vi "VFH-read_file-R140_waterfile.vi"(8 "error in (no error)":errorcluster) -> (0 "error out":errorcluster, 2 "Array":T1[](array[typedef]))   [LabVIEW 2020, in "VFH-VNA_File_Handler.lvlib"]
uses:
  VFH-VNA_File_Handler.lvlib
  VFH-file_cluster-r140_water.ctl
  <vilib>/addons/_office/excel.llb/Excel Get Data ([dbl]).vi
  <vilib>/Utility/NIReport.llb/NI_report.lvclass
  <vilib>/Utility/NIReport.llb/Excel/NI_Excel.lvclass
  <vilib>/addons/_office/NI_ReportGenerationToolkit.lvlib
panel:
  out "XY Graph":cluster{"Frequency":dbl[], "Permativity'":dbl[]}(graph)
  out "handled Data":dbl[](array[numeric])
  out "Waveform Graph 2":dbl[](graph)
  out "Waveform Graph":dbl[](graph)
  out "Sheet 1 Data":dbl[][](array[numeric]) format="%.2f"
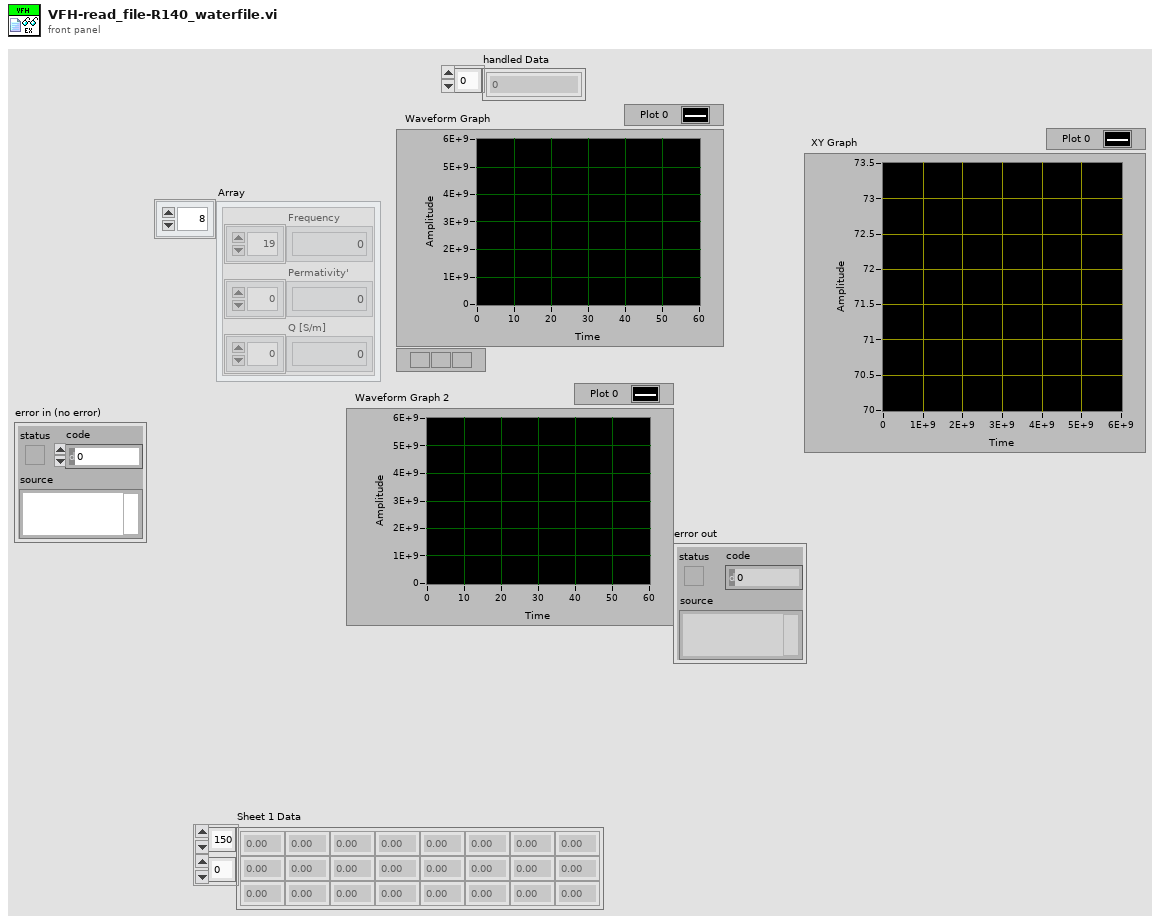
[diagram p1: front panel]
types:
  T1 = typedef "VFH-VNA_File_Handler.lvlib/VFH-file_cluster-r140_water.ctl" = cluster{"Frequency":dbl[], "Permativity'":dbl[], "Q [S/m]":dbl[]}
  T2 = enum16{"Standard Report", "HTML", "Word", "Excel"}
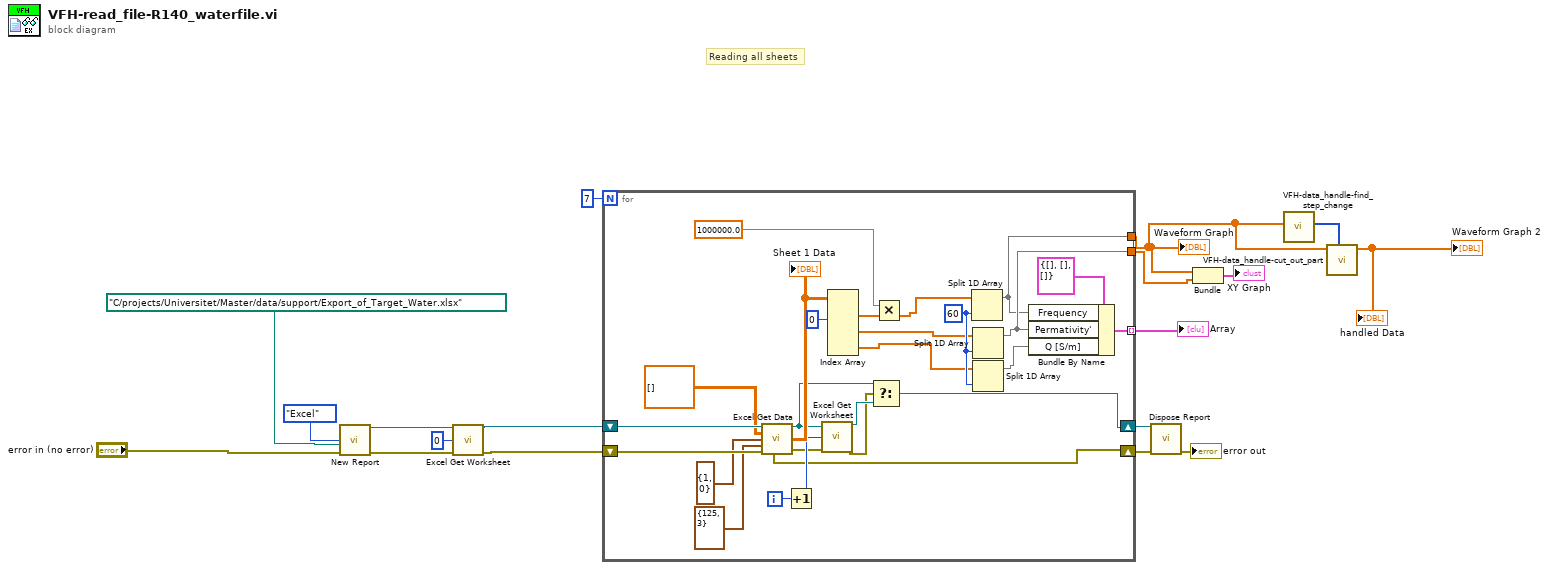
[diagram p0: block diagram]
diagram:
  # "Reading all sheets"
  n1 = call <vilib>:"New Report.vi"("report type"=T2."Excel", "template (empty)"=path "C:/projects/Universitet/Master/data/support/Export_of_Target_Water.xlsx" ("file path (dialog if empty)"), "error in (no error)"="error in (no error)") -> ("report out"=w12:refnum<class "NI_report.lvclass">, "error out"=w11:errorcluster)  [unwired: 3 in, 8 out]
  n2 = call <vilib>:"Excel Get Worksheet.vi"("report in"=w12, "worksheet index (0)"=0, "error in (no error)"=w11) -> ("report out"=w9:refnum<class "NI_report.lvclass">, "error out"=w8:errorcluster)  [unwired: 11 out]
  n3 = for {
    N: 7 -> [_]
    shift-right: [w31] -> w17
    shift-left: w9 -> [w43]
    shift-right: [w34] -> w16
    shift-left: w8 -> [w41]
    tunnel: [w28] -> w5 mode=indexing
    tunnel: [w19] -> w3
    tunnel: [w20] -> w2
    i -> [w36]
    w24 = 60 ("index")
    n4 = call-poly <vilib>:"Excel Get Data.vi"("report in"=w43, "data type"=dbl[][] [], "start (-1, -1)"=cluster{"row":i32, "column":i32} {"row"=1, "column"=0}, "end (-1, -1)"=cluster{"row":i32, "column":i32} {"row"=125, "column"=3}, "error in (no error)"=w41) -> ("report out"=w33:refnum<class "NI_report.lvclass">, "data"=w37:dbl[][], "error out"=w34:errorcluster)  [unwired: 8 out]
    "Sheet 1 Data" <- w37
    n5 = Increment(x=w36) -> (x+1=w35:i32)
    n6 = call <vilib>:"Excel Get Worksheet.vi"("report in"=w33, "worksheet index (0)"=w35, "error in (no error)"=w34) -> ("report out"=w32:refnum<class "NI_report.lvclass">, "error out"=w30:errorcluster)  [unwired: 11 out]
    n7 = Index Array(array=w37, index (col) #1=0 ("disabled index (col)")) -> (element #1=w27:dbl[], element #2=w23:dbl[], element #3=w21:dbl[])  [unwired: 5 in]
    n8 = Select(t=w33, s=w30, f=w32) -> (s? t:f=w31:refnum<class "NI_report.lvclass">)
    n9 = Multiply(x=1000000.0, y=w27) -> (x*y=w25:dbl[])
    n10 = Split 1D Array(array=w25, index=w24) -> (first subarray=w19:dbl[])  [unwired: 1 out]
    n11 = Split 1D Array(array=w23, index=w24) -> (first subarray=w20:dbl[])  [unwired: 1 out]
    n12 = Split 1D Array(array=w21, index=w24) -> (first subarray=w22:dbl[])  [unwired: 1 out]
    n13 = Bundle By Name(cluster=T1 {"Frequency"=[], "Permativity'"=[], "Q [S/m]"=[]} ("output cluster"), "Frequency"=w19, "Permativity'"=w20, "Q [S/m]"=w22) -> (w28:T1)
  }
  "Array" <- w5
  "Waveform Graph" <- w3
  n14 = call-dynamic "Dispose Report.vi"("report in"=w17, "error in (no error)"=w16) -> ("error out"=→"error out":errorcluster)  [unwired: 3 in, 10 out]
  n15 = Bundle(w3, w2) -> (→"XY Graph":cluster{dbl[], dbl[]})  [unwired: 1 in]
  n16 = call "VFH-data_handle-find_step_change.vi"("data"=w3) -> ("step points"=w7:i32[])  [unwired: 10 in]
  n17 = call "VFH-data_handle-cut_out_part.vi"("Start and stop"=w7, "data"=w3) -> ("handled Data"=→"Waveform Graph 2" →"handled Data":dbl[])  [unwired: 8 in, 1 out]
